vi "read_data.vi"(8 "error in (no error)":errorcluster, 11 "MG090622IMAQCamera in":refnum<class "DAQ_MG090622Camera.lvclass">) -> (0 "error out":errorcluster, 2 "finished?":bool, 3 "MG090622IMAQCamera out":refnum<class "DAQ_MG090622Camera.lvclass">, 4 "buffer overflow?":bool)   [LabVIEW 2010, in "DAQ_MG090622Camera.lvclass"]
uses:
  DAQ_MG090622Camera.lvclass
  common/classes/Image/Image/Image.lvclass
  <vilib>/vision/NI_Vision_Development_Module.lvlib
  common/classes/ErrorController/ErrorController/ErrorController.lvclass
  <vilib>/vision/driver/NI_Vision_Acquisition_Software.lvlib
panel:
  out "image":T1(plugin-control)
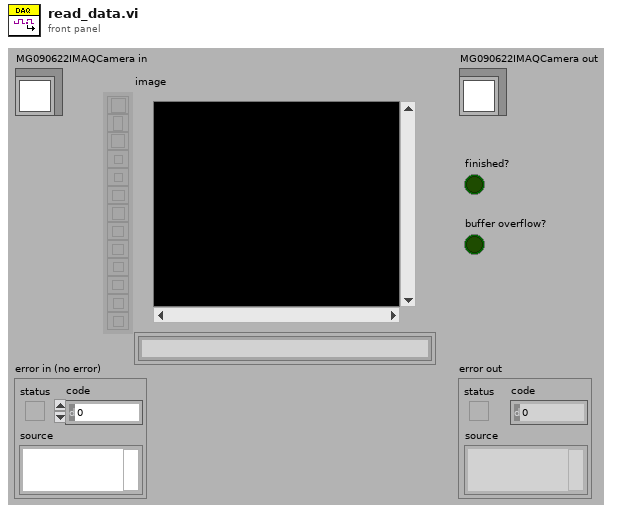
[diagram p1: front panel]
types:
  T1 = typedef "IMAQ Image.ctl" = refnum<image>
  T2 = typedef "DAQ_MG090622Camera.lvclass/camera_type_enum.ctl" = enum16{"gray scale", "RGB"}
  T3 = typedef "DAQ_MG090622Camera.lvclass/connection_type_enum.ctl" = enum16{"IEEE 1394 (FireWire)", "USB", "GigE", "CameraLink"}
  T4 = typedef "IMAQdx.ctl" = refnum<k21>
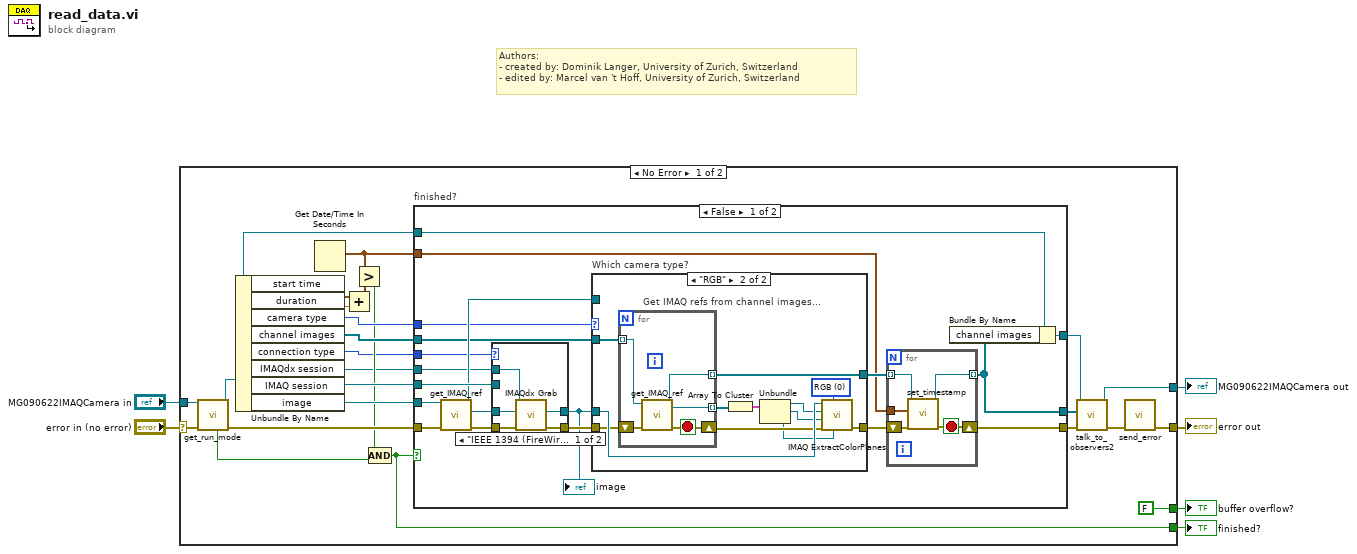
[diagram p0: block diagram]
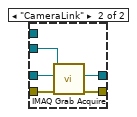
[diagram p2: hidden frame]
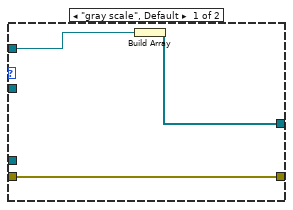
[diagram p3: hidden frame]
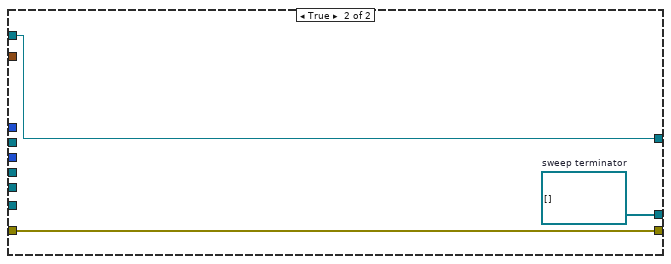
[diagram p4: hidden frame]
diagram:
  # "Authors: \n- created by: Dominik Langer, University of Zurich, Switzerland\n- edited by: Marcel van 't Hoff, University of Zurich, Switzerland"
  n1 = case shown="No Error" "error in (no error)" {
    selector: "error in (no error)" -> [w23 w89]
    tunnel: [w15 w89] -> w4
    tunnel: [w8 w88] -> w3
    tunnel: "MG090622IMAQCamera in" -> [w21 w88]
    tunnel: [w17 _] -> w2
    tunnel: [FALSE _] -> w1
    frame No Error {
      n2 = call-dynamic "get_run_mode.vi"("error in (no error)"=w23, "GenericPlugin in"=w21) -> ("error out"=w22:errorcluster, "GenericPlugin out"=w9:refnum<class "DAQ_MG090622Camera.lvclass">, "is NOT free run?"=w18:bool)  [unwired: 5 in, 2 out]
      n3 = Unbundle By Name(w9) -> ("start time"=w19:timestamp, "duration"=w26:dbl[unit], "camera type"=w27:T2, "channel images"=w28:refnum<class "Image.lvclass">[], "connection type"=w14:T3, "IMAQdx session"=w13:T4, "IMAQ session"=w29:refnum<k11>, "image"=w30:refnum<class "Image.lvclass">)
      n4 = Get Date/Time In Seconds() -> (seconds since 1Jan1904=w24:timestamp)
      n5 = Add(x=w19, y=w26) -> (x+y=w25:timestamp)
      n6 = Greater?(x=w24, y=w25) -> (0:w16:bool)
      n7 = Compound Arithmetic op=AND(w16, w18) -> (w17:bool)
      n8 = case "finished?" shown="False" w17 {
        tunnel: w30 -> [w49 _]
        tunnel: w29 -> [w48 _]
        tunnel: w28 -> [w43 _]
        tunnel: w27 -> [w42 _]
        tunnel: w24 -> [w39 _]
        tunnel: w22 -> [w38 w87]
        tunnel: [w34 w87] -> w11
        tunnel: w14 -> [w36 _]
        tunnel: w13 -> [w35 _]
        tunnel: [w31 w86] -> w10
        tunnel: w9 -> [w33 w85]
        tunnel: [w32 w85] -> w7
        frame False {
          n9 = call-dynamic "get_IMAQ_ref.vi"("error in (no error)"=w38, "Image.lvclass in"=w49) -> ("error out"=w46:errorcluster, "Image"=w47:T1, "Image.lvclass out"=w44:refnum<class "Image.lvclass">)  [unwired: 7 out]
          n10 = case shown="\"IEEE 1394 (FireWire)\", Default" w36 {
            tunnel: w48 -> [_ w59]
            tunnel: w47 -> [w52 w58]
            tunnel: w46 -> [w54 w57]
            tunnel: [w53 w56] -> w45
            tunnel: [w51 w55] -> w37
            tunnel: w35 -> [w50 _]
            frame "IEEE 1394 (FireWire)", Default {
              n11 = call <vilib>:"IMAQdx Grab.vi"("error in"=w54, "Image In"=w52, "Session In"=w50) -> ("error out"=w53:errorcluster, "Image Out"=w51:T1)  [unwired: 5 in, 2 out]
            }
            frame "CameraLink" {
              n12 = call <vilib>:"IMAQ Grab Acquire.vi"("error in (no error)"=w57, "Image In"=w58, "IMAQ Session In"=w59) -> ("error out"=w56:errorcluster, "Image Out"=w55:T1)  [unwired: 1 in, 6 out]
            }
          }
          "image" <- w37
          n13 = case "Which camera type?" shown="\"RGB\"" w42 {
            tunnel: [w67 w78] -> w40
            tunnel: w45 -> [w66 w75]
            tunnel: w44 -> [w65 _]
            tunnel: w37 -> [_ w77]
            tunnel: w43 -> [_ w76]
            tunnel: [w66 w74] -> w41
            frame "gray scale", Default {
              n14 = Build Array(w65) -> (w67:refnum<class "Image.lvclass">[])
            }
            frame "RGB" {
              w68 = u16 0 items=["RGB", "HSL", "HSV", "HSI"] ("Color Mode")
              n15 = for "Get IMAQ refs from channel images..." {
                tunnel: [w84] -> w79 mode=indexing
                tunnel: [w83] -> w78 mode=indexing
                tunnel: w76 -> [w82] mode=indexing
                shift-right: [w80] -> w73
                shift-left: w75 -> [w81]
                stop <- w80 stop-if-true
                n16 = call-dynamic "get_IMAQ_ref.vi"("error in (no error)"=w81, "Image.lvclass in"=w82) -> ("error out"=w80:errorcluster, "Image"=w84:T1, "Image.lvclass out"=w83:refnum<class "Image.lvclass">)  [unwired: 7 out]
              }
              n17 = Array To Cluster(array=w79) -> (cluster=w72:cluster{"[0]":T1, "[1]":T1, "[2]":T1})
              n18 = Unbundle(w72) -> ("[0]"=w71:T1, "[1]"=w70:T1, "[2]"=w69:T1)
              n19 = call "IMAQ ExtractColorPlanes"("Blue or Luma or Val or Inten Plane"=w69, "Color Mode"=w68, "error in (no error)"=w73, "Green or Sat Plane"=w70, "Red or Hue Plane"=w71, "Image Src"=w77) -> ("error out"=w74:errorcluster)  [unwired: 5 out]
            }
          }
          n20 = for {
            tunnel: w40 -> [w62] mode=indexing
            shift-right: [w60] -> w34
            shift-left: w41 -> [w63]
            tunnel: w39 -> [w64]
            tunnel: [w61] -> w31 mode=indexing
            stop <- w60 stop-if-true
            n21 = call-dynamic "set_timestamp.vi"("error in (no error)"=w63, "timestamp"=w64, "Image.lvclass in"=w62) -> ("error out"=w60:errorcluster, "Image.lvclass out"=w61:refnum<class "Image.lvclass">)  [unwired: 7 out]
          }
          n22 = Bundle By Name(cluster=w33, "channel images"=w31) -> (w32:refnum<class "DAQ_MG090622Camera.lvclass">)
        }
        frame True {
          w86 = refnum<class "Image.lvclass">[] []  # sweep terminator
        }
      }
      n23 = call-dynamic "talk_to_observers2.vi"("error in (no error)"=w11, "image (channels)"=w10, "GenericToplevelComponent in"=w7) -> ("error out"=w12:errorcluster, "GenericToplevelComponent out"=w8:refnum<class "DAQ_MG090622Camera.lvclass">)  [unwired: 7 in]
      n24 = call "send_error.vi"("error in (no error)"=w12) -> ("error out"=w15:errorcluster)  [unwired: 10 in]
    }
    frame Error {
    }
  }
  "error out" <- w4
  "MG090622IMAQCamera out" <- w3
  "finished?" <- w2
  "buffer overflow?" <- w1
